vi "Indicators.vi"(0 "Overlimit Value":bool, 1 "Underlimit Value":bool) -> ()   [LabVIEW 2021]
uses:
  <vilib>/Utility/error.llb/Error Cluster From Error Code.vi
  <vilib>/myRIO/Common/Instrument Driver Framework/myRIO v1.0/DIO/vis/myRIO v1.0 Write DIO.vi
  <vilib>/myRIO/Instrument Drivers/Onboard IO/DIO/DIO.lvlib
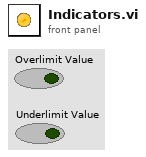
[diagram p1: front panel]
types:
  T1 = typedef "DIO.lvlib/DIO Reference.ctl" = cluster{"myRIO Reference":T2, "DIO Channels List":T6}
  T2 = typedef "myRIO Generic Hardware Reference.ctl" = cluster{"myRIO Model":T3, "myRIO Hardware Reference":T4}
  T3 = typedef "Hardware Version Enum.ctl" = enum16{"Unknown", "myRIO-1900", "myRIO-1950", "roboRIO", "NI ELVIS RIO CM", "ELVIS III"}
  T4 = typedef "myRIO v1.0 Reference.ctl" = cluster{"Generic FPGA Reference":T5, "Allow multiple opens":bool}
  T5 = typedef "Generic FPGA Reference.ctl" = refnum<k20>
  T6 = typedef "DIO Channels List.ctl" = T7[]
  T7 = typedef "DIO Channels Enum.ctl" = enum16{"Not Connected", "C/DIO0", "C/DIO1", "C/DIO2", "C/DIO3", "C/DIO4", "C/DIO5", "C/DIO6", "C/DIO7", "A/DIO0", "A/DIO1", "A/DIO2", "A/DIO3", "A/DIO4", "A/DIO5", "A/DIO6", "A/DIO7", "A/DIO8", "A/DIO9", "A/DIO10", "A/DIO11", "A/DIO12", "A/DIO13", "A/DIO14", "A/DIO15", "A/DIO16", "A/DIO17", "A/DIO18", "A/DIO19", "B/DIO0", "B/DIO1", "B/DIO2", "B/DIO3", "B/DIO4", "B/DIO5", "B/DIO6", "B/DIO7", "B/DIO8", "B/DIO9", "B/DIO10", "B/DIO11", "B/DIO12", "B/DIO13", "B/DIO14", "B/DIO15", "B/DIO16", "B/DIO17", "B/DIO18", "B/DIO19", "LED0", "LED1", "LED2", "LED3", "Button0", "DIO/DIO0", "DIO/DIO1", "DIO/DIO2", "DIO/DIO3", "DIO/DIO4", "DIO/DIO5", "DIO/DIO6", "DIO/DIO7", "DIO/DIO8", "DIO/DIO9", "SPI/CS0", "SPI/CS1", "SPI/CS2", "SPI/CS3", "LED RADIO (Green)", "LED RADIO (Red)", "LED COMM (Green)", "LED COMM (Red)", "LED MODE (Green)", "LED MODE (Red)"}
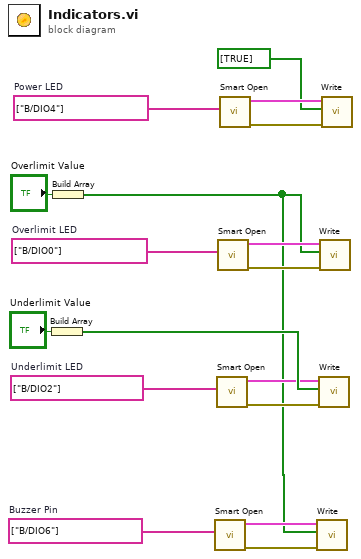
[diagram p0: block diagram]
diagram:
  w6 = tag[] ["B/DIO0"]  # Overlimit LED
  w9 = tag[] ["B/DIO4"]  # Power LED
  w12 = tag[] ["B/DIO6"]  # Buzzer Pin
  w17 = tag[] ["B/DIO2"]  # Underlimit LED
  n1 = Build Array("Underlimit Value") -> (w16:bool[])
  n2 = Build Array("Overlimit Value") -> (w1:bool[])
  n3 = call <vilib>:"Smart Open.vi"("Channel Names"=w12) -> ("error out"=w10:errorcluster, "DIO Ref Out"=w11:T1)  [unwired: 9 in]
  n4 = call <vilib>:"Smart Open.vi"("Channel Names"=w17) -> ("error out"=w13:errorcluster, "DIO Ref Out"=w14:T1)  [unwired: 9 in]
  n5 = call <vilib>:"Smart Open.vi"("Channel Names"=w6) -> ("error out"=w3:errorcluster, "DIO Ref Out"=w4:T1)  [unwired: 9 in]
  n6 = call <vilib>:"Smart Open.vi"("Channel Names"=w9) -> ("error out"=w7:errorcluster, "DIO Ref Out"=w8:T1)  [unwired: 9 in]
  n7 = call <vilib>:"Write.vi"("error in (no error)"=w10, "Values"=w1, "DIO Ref In"=w11) -> ()  [unwired: 6 in, 2 out]
  n8 = call <vilib>:"Write.vi"("error in (no error)"=w13, "Values"=w16, "DIO Ref In"=w14) -> ()  [unwired: 6 in, 2 out]
  n9 = call <vilib>:"Write.vi"("error in (no error)"=w3, "Values"=w1, "DIO Ref In"=w4) -> ()  [unwired: 6 in, 2 out]
  n10 = call <vilib>:"Write.vi"("error in (no error)"=w7, "Values"=bool[] [TRUE], "DIO Ref In"=w8) -> ()  [unwired: 6 in, 2 out]
